vi "Read Multi-Channel Waveform.vi"(8 "error in (no error)":errorcluster, 10 "Channels":T1[](array[typedef]), 11 "PXIe5105 in":refnum<class "PXIe5105.lvclass">) -> (0 "error out":errorcluster, 2 "Waveform":waveform(dbl)[](graph), 3 "PXIe5105 out":refnum<class "PXIe5105.lvclass">)   [LabVIEW 2018, in "PXIe5105.lvlib" / "PXIe5105.lvclass"]
doc: "This Override method is used to initiate multi-channel waveform acquisition. Select targeted channels at the 'Channels' control and output waveform data to the 'Waveform' indicator."
uses:
  PXIe5105.lvclass
  PPLs/Oscilloscope/Parent/Oscilloscope.lvlibp/Custom Controls/Analog Channels.ctl
  PXIe5105.lvclass/PXIe5105.ctl
  <instrlib>/niScope/Acquire/Fetch/niScope Multi Fetch WDT.vi
  PPLs/Oscilloscope/Parent/Oscilloscope.lvlibp
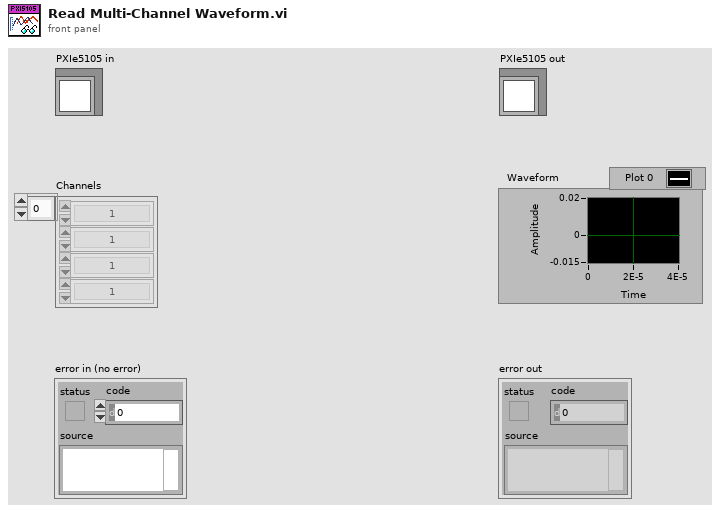
[diagram p1: front panel]
types:
  T1 = typedef "Oscilloscope.lvlibp/Analog Channels.ctl" = enum16{"1", "2", "3", "4", "5", "6", "7", "8", "9", "10", "11", "12", "13", "14", "15", "16"}
  T2 = typedef "niScope timestamp type.ctl" = i32
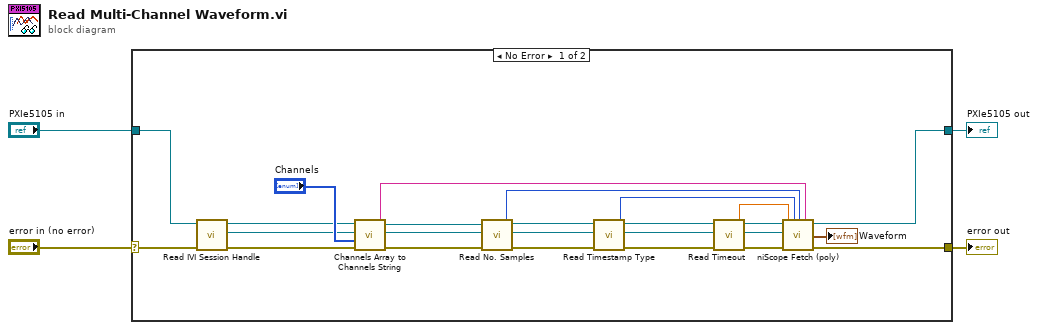
[diagram p0: block diagram]
diagram:
  n1 = case shown="No Error" "error in (no error)" {
    selector: "error in (no error)" -> [w19 w26]
    tunnel: [w5 w26] -> w3
    tunnel: [w14 w25] -> w2
    tunnel: "PXIe5105 in" -> [w21 w25]
    frame No Error {
      n2 = call "Read IVI Session Handle.vi"("error in (no error)"=w19, "PXIe5105 in"=w21) -> ("error out"=w18:errorcluster, "IVI Session Handle"=w8:refnum<k15>, "PXIe5105 out"=w20:refnum<class "PXIe5105.lvclass">)  [unwired: 7 in]
      n3 = call "Channels Array to Channels String.vi"("error in (no error)"=w18, "Channel(s) Array"="Channels", "PXIe5105 in"=w20) -> ("error out"=w24:errorcluster, "Channels String"=w12:string, "PXIe5105 out"=w23:refnum<class "PXIe5105.lvclass">)  [unwired: 6 in]
      n4 = call "Read No. Samples.vi"("error in (no error)"=w24, "PXIe5105 in"=w23) -> ("error out"=w13:errorcluster, "No. Samples"=w11:i32, "PXIe5105 out"=w15:refnum<class "PXIe5105.lvclass">)  [unwired: 7 in]
      n5 = call "Read Timestamp Type.vi"("error in (no error)"=w13, "PXIe5105 in"=w15) -> ("error out"=w17:errorcluster, "timestamp type"=w10:T2, "PXIe5105 out"=w16:refnum<class "PXIe5105.lvclass">)  [unwired: 7 in]
      n6 = call "Read Timeout.vi"("error in (no error)"=w17, "PXIe5105 in"=w16) -> ("error out"=w7:errorcluster, "Timeout"=w9:dbl, "PXIe5105 out"=w14:refnum<class "PXIe5105.lvclass">)  [unwired: 7 in]
      n7 = call-poly <instrlib>:"niScope Fetch (poly).vi"("timestamp Type"=w10, "timeout"=w9, "error in"=w7, "numSamples"=w11, "channels"=w12, "instrument handle"=w8) -> ("error out"=w5:errorcluster, "wfm"=→"Waveform":waveform(dbl)[])  [unwired: 2 in, 2 out]
    }
    frame Error {
    }
  }
  "error out" <- w3
  "PXIe5105 out" <- w2
